vi "To Variant.vi"(8 "Error In":errorcluster, 11 "TD Bool A":refnum<class "1D Bool.lvclass">) -> (0 "Error Out":errorcluster, 2 "Variant":variant)   [LabVIEW 2017, in "Tree API.lvlib" / "1D Bool.lvclass"]
doc: "Dynamic dispatch interface for conversion of Tree Data classes to variant LV data."
uses:
  1D Bool.lvclass
  Tree Data/Tree Data.lvclass
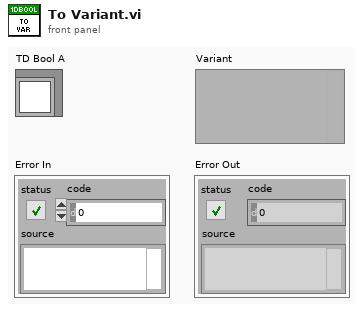
[diagram p1: front panel]
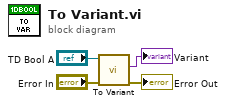
[diagram p0: block diagram]
diagram:
  n1 = call-parent "To Variant.vi"("Error In"="Error In", "Tree Data"="TD Bool A") -> ("Error Out"=→"Error Out":errorcluster, "Variant"=→"Variant":variant)  [unwired: 8 in]
